vi "Procces coin.vi"(8 "error in (no error)":errorcluster, 10 "Coins":T1, 11 "USD Actor in":refnum<class "USD Actor.lvclass">) -> (0 "error out":errorcluster, 3 "USD Actor out":refnum<class "USD Actor.lvclass">)   [LabVIEW 2020, in "USD Actor.lvlib" / "USD Actor.lvclass"]
uses:
  USD Actor.lvclass
  C:/Program Files (x86)/National Instruments/LabVIEW 2020/vi.lib/ActorFramework/Actor/Actor.lvclass
  <vilib>/ActorFramework/Actor/Actor.lvclass/Actor.ctl
  USD Actor.lvclass/USD Actor.ctl
  UI Actor Messages/Credit Update Msg/Credit Update Msg.lvclass/Credit Update Msg.ctl
  <vilib>/ActorFramework/Message Enqueuer/Message Enqueuer.lvclass/Message Enqueuer.ctl
  <vilib>/ActorFramework/Message Enqueuer/Enqueue.vi
  UI Actor Messages/Credit Update Msg/Credit Update Msg.lvclass
  C:/Program Files (x86)/National Instruments/LabVIEW 2020/vi.lib/ActorFramework/Message/Message.lvclass
  <vilib>/ActorFramework/Message Priority Queue/Priority Enqueue.vi
  <vilib>/ActorFramework/Actor/Actor.lvclass
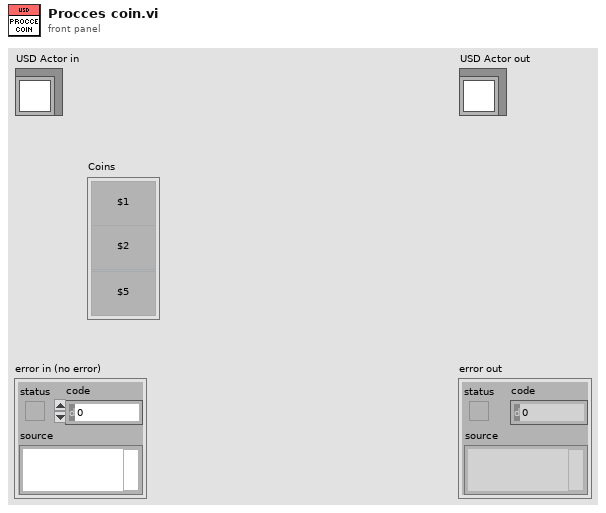
[diagram p1: front panel]
types:
  T1 = cluster{"Button":bool, "Button 2":bool, "Button 3":bool}
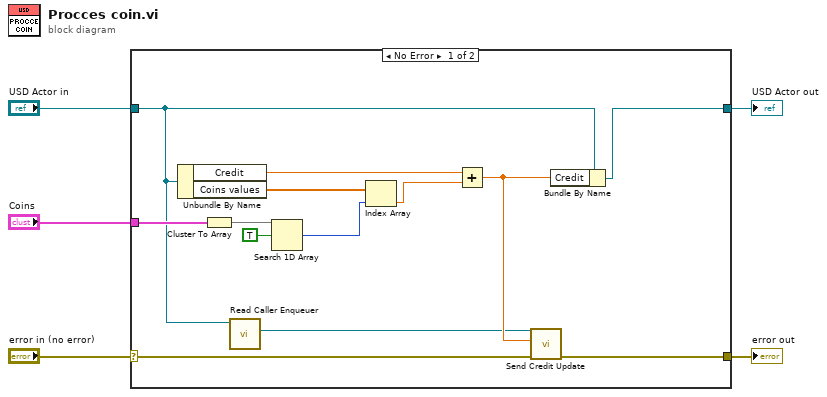
[diagram p0: block diagram]
diagram:
  n1 = case shown="No Error" "error in (no error)" {
    selector: "error in (no error)" -> [w8 w20]
    tunnel: [w7 w20] -> w4
    tunnel: [w11 w19] -> w2
    tunnel: "USD Actor in" -> [w10 w19]
    tunnel: "Coins" -> [w16 _]
    frame No Error {
      n2 = Unbundle By Name(w10) -> ("Credit"=w13:dbl, "Coins values"=w14:dbl[])
      n3 = Cluster To Array(cluster=w16) -> (array=w18:bool[])
      n4 = call <vilib>:"Read Caller Enqueuer.vi"("Actor"=w10) -> ("Caller Enqueuer"=w6:refnum<class "Message Enqueuer.lvclass">)  [unwired: 10 in]
      n5 = Search 1D Array(1D array=w18, element=TRUE) -> (index of element=w15:i32)  [unwired: 1 in]
      n6 = Index Array(array=w14, index=w15) -> (element=w12:dbl)
      n7 = Add(x=w13, y=w12) -> (x+y=w9:dbl)
      n8 = call "Send Credit Update.vi"("error in (no error)"=w8, "Credit"=w9, "Message Enqueuer"=w6) -> ("error out"=w7:errorcluster)  [unwired: 7 in, 1 out]
      n9 = Bundle By Name(cluster=w10, "Credit"=w9) -> (w11:refnum<class "USD Actor.lvclass">)
    }
    frame Error {
    }
  }
  "error out" <- w4
  "USD Actor out" <- w2
